vi "toXml.vi"(8 "error in (no error)":errorcluster, 11 "DigitalOutput in":refnum<class "DigitalOutput.lvclass">) -> (0 "error out":errorcluster, 2 "Array":string[](array[string]), 3 "DigitalOutput out":refnum<class "DigitalOutput.lvclass">)   [LabVIEW 2011, in "Hardware.lvlib" / "Channels.lvlib" / "DigitalOutput.lvclass"]
uses:
  DigitalOutput.lvclass
  DigitalOutput.lvclass/DigitalOutput.ctl
panel:
  out "Array 2":string[](array[string])
  out "output cluster":T1
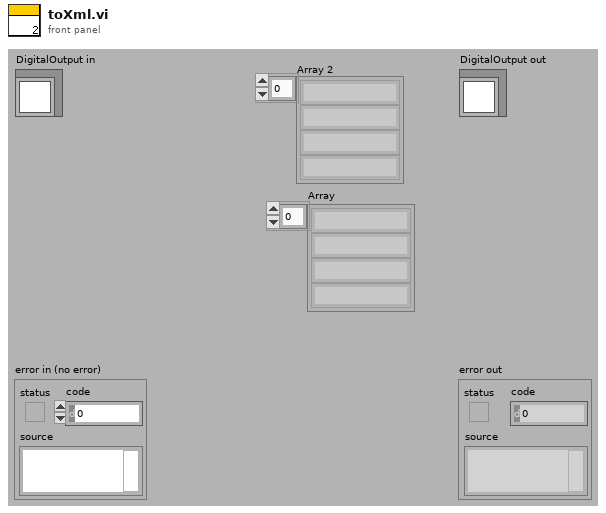
[diagram p1: front panel]
types:
  T1 = cluster{"name":string, "Physical Channels":string, "Timing":cluster{"Master Clock source":string, "Master Clock rate":dbl, "Start trigger line":string, "Scan rate":dbl, "Stop trigger line":string, "Sample Number":dbl}, "Routings":cluster{"Master Clock Route":string[]}, "Data":cluster{"Timestamps ms":dbl[], "Bitmap":bool[][]}}
  T2 = cluster{"Master Clock source":string, "Master Clock rate":dbl, "Start trigger line":string, "Scan rate":dbl, "Stop trigger line":string, "Sample Number":dbl}
  T3 = cluster{"Timestamps ms":dbl[], "DataPerChannel":dbl[][]}
  T4 = cluster{"name":string, "Physical Channels":string, "Timing":cluster{"Master Clock source":string, "Master Clock rate":dbl, "Start trigger line":string, "Scan rate":dbl, "Stop trigger line":string, "Sample Number":dbl}, "Routings":cluster{"Master Clock Route":string[]}, "Data":cluster{"Timestamps ms":dbl[], "DataPerChannel":dbl[][]}}
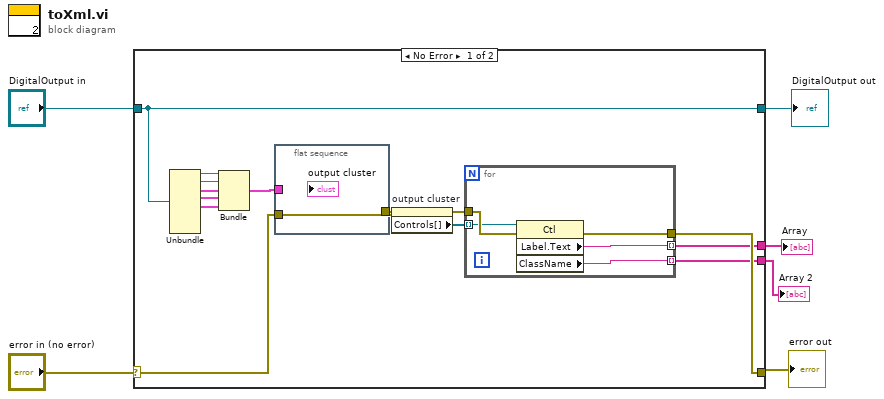
[diagram p0: block diagram]
diagram:
  n1 = case shown="No Error" "error in (no error)" {
    selector: "error in (no error)" -> [w10 w28]
    tunnel: [w12 w28] -> w3
    tunnel: [w20 w27] -> w4
    tunnel: "DigitalOutput in" -> [w20 w27]
    tunnel: [w8 _] -> w2
    tunnel: [w7 _] -> w1
    frame No Error {
      n2 = Unbundle(w20) -> (w19:string, w18:string, w17:T2, w16:cluster{"Master Clock Route":string[]}, w15:T3)  [unwired: 3 out]
      n3 = Bundle("name"=w19, "Physical Channels"=w18, "Timing"=w17, "Routings"=w16, "Data"=w15) -> (w11:T4)  [unwired: 1 in]
      n4 = flat-sequence {
        tunnel: w11 -> [_]
        tunnel: w10 -> [w21]
        tunnel: [w21] -> w9
        frame #0 {
        }
      }
      n5 = property on="output cluster" class="Clust (strict)"(error in=w9) -> (error out=w13:errorcluster, "Controls[]"=w14:refnum<vi>[])  [unwired: 1 in, 1 out]
      n6 = for {
        tunnel: w14 -> [w23] mode=indexing
        tunnel: w13 -> [w26]
        tunnel: [w25] -> w12
        tunnel: [w24] -> w8 mode=indexing
        tunnel: [w22] -> w7 mode=indexing
        n7 = property class="Ctl"(reference=w23, error in=w26) -> (error out=w25:errorcluster, "Label.Text"=w24:string, "ClassName"=w22:string)  [unwired: 1 out]
      }
    }
    frame Error {
    }
  }
  "error out" <- w3
  "DigitalOutput out" <- w4
  "Array" <- w2
  "Array 2" <- w1
